vi "Test Data Type.vi"() -> ()   [LabVIEW 2017]
uses:
  <userlib>/_NEVSTOP/Communicable State Machine(CSM)/Communicable State Machine.lvlib
panel:
  out "String 14":string
  out "String 13":string
  out "String 12":string
  out "String 11":string
  out "String 10":string
  out "String 9":string
  out "String 8":string
  out "String 7":string
  out "String 6":string
  out "String 5":string
  out "String 4":string
  out "String 3":string
  out "String 2":string
  out "String":string
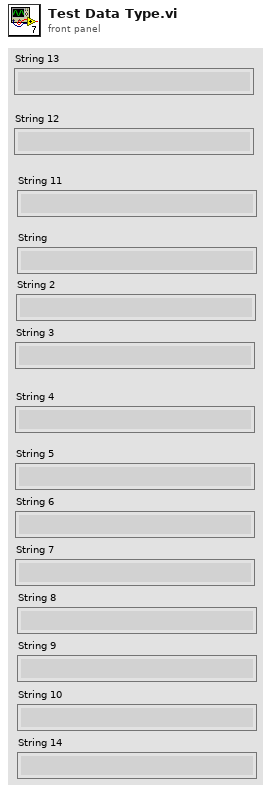
[diagram p1: front panel]
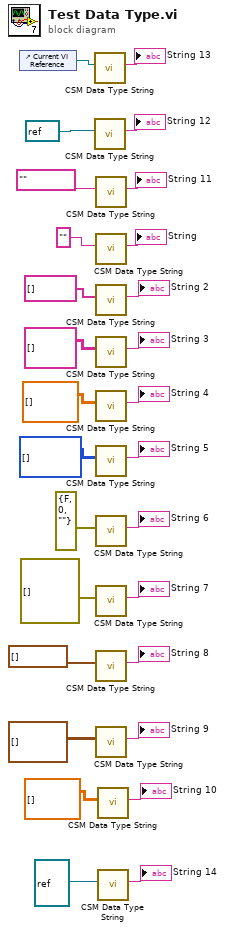
[diagram p0: block diagram]
diagram:
  n1 = control-ref of="Current VI Reference"() -> (w3:refnum<vi>)
  n2 = call <userlib>:"CSM Data Type String.vi"("Data"=w3) -> ("Data Type String"=→"String 13":string)  [unwired: 10 in]
  n3 = call <userlib>:"CSM Data Type String.vi"("Data"=refnum<k21> refnum) -> ("Data Type String"=→"String 12":string)  [unwired: 10 in]
  n4 = call <userlib>:"CSM Data Type String.vi"("Data"=tag "") -> ("Data Type String"=→"String 11":string)  [unwired: 10 in]
  n5 = call <userlib>:"CSM Data Type String.vi"("Data"="") -> ("Data Type String"=→"String":string)  [unwired: 10 in]
  n6 = call <userlib>:"CSM Data Type String.vi"("Data"=string[] []) -> ("Data Type String"=→"String 2":string)  [unwired: 10 in]
  n7 = call <userlib>:"CSM Data Type String.vi"("Data"=string[][] []) -> ("Data Type String"=→"String 3":string)  [unwired: 10 in]
  n8 = call <userlib>:"CSM Data Type String.vi"("Data"=dbl[][] []) -> ("Data Type String"=→"String 4":string)  [unwired: 10 in]
  n9 = call <userlib>:"CSM Data Type String.vi"("Data"=i32[][] []) -> ("Data Type String"=→"String 5":string)  [unwired: 10 in]
  n10 = call <userlib>:"CSM Data Type String.vi"("Data"=errorcluster {"status"=FALSE, "code"=0, "source"=""} ("error in (no error)")) -> ("Data Type String"=→"String 6":string)  [unwired: 10 in]
  n11 = call <userlib>:"CSM Data Type String.vi"("Data"=errorcluster[] [] ("error in (no error)")) -> ("Data Type String"=→"String 7":string)  [unwired: 10 in]
  n12 = call <userlib>:"CSM Data Type String.vi"("Data"=waveform(dbl)[] [] ("error in (no error)")) -> ("Data Type String"=→"String 8":string)  [unwired: 10 in]
  n13 = call <userlib>:"CSM Data Type String.vi"("Data"=waveform(dbl)[][] [] ("error in (no error)")) -> ("Data Type String"=→"String 9":string)  [unwired: 10 in]
  n14 = call <userlib>:"CSM Data Type String.vi"("Data"=ext[][] []) -> ("Data Type String"=→"String 10":string)  [unwired: 10 in]
  n15 = call <userlib>:"CSM Data Type String.vi"("Data"=refnum<vi> refnum ("Current VI's reference")) -> ("Data Type String"=→"String 14":string)  [unwired: 10 in]
